vi "Main Auton Script XML Converter.vi"() -> ()   [LabVIEW 2014]
panel:
  in  "Array":string[][](array[string])
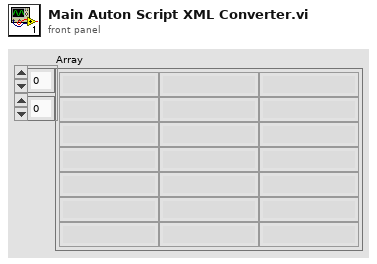
[diagram p1: front panel]
types:
  T1 = enum16{"open", "replace", "create", "open or create", "replace or create", "replace or create with confirmation"}
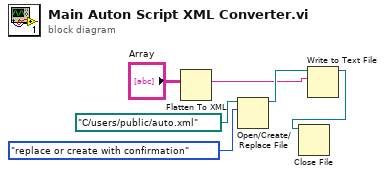
[diagram p0: block diagram]
diagram:
  n1 = Flatten To XML(anything="Array") -> (xml string=w1:string)
  n2 = Open/Create/Replace File(file path (use dialog)=path "C:/users/public/auto.xml", operation (0:open)=T1."replace or create with confirmation") -> (refnum out=w3:refnum<file>)  [unwired: 4 in, 2 out]
  n3 = Write to Text File(file (use dialog)=w3, text=w1) -> (refnum out=w2:refnum<file>)  [unwired: 2 in, 2 out]
  n4 = Close File(refnum=w2) -> ()  [unwired: 1 in, 2 out]
